vi "CLD 1 Elapsed Time Express Front Panel.vi"() -> ()   [LabVIEW 2009]
doc: "LabVIEW CLD-Übung 1"
panel:
  out "Fehler (Ausgang)":errorcluster
  in  "Fehler (Eingang)":errorcluster
  out "Verstrichene Zeit":string
  out "Zeit ist verstrichen":bool
  in  "Autom. zurücksetzen":bool
  in  "Zurücksetzen-Schaltfläche":bool
  in  "VI anhalten":bool
  in  "Zielzeit (s)":dbl
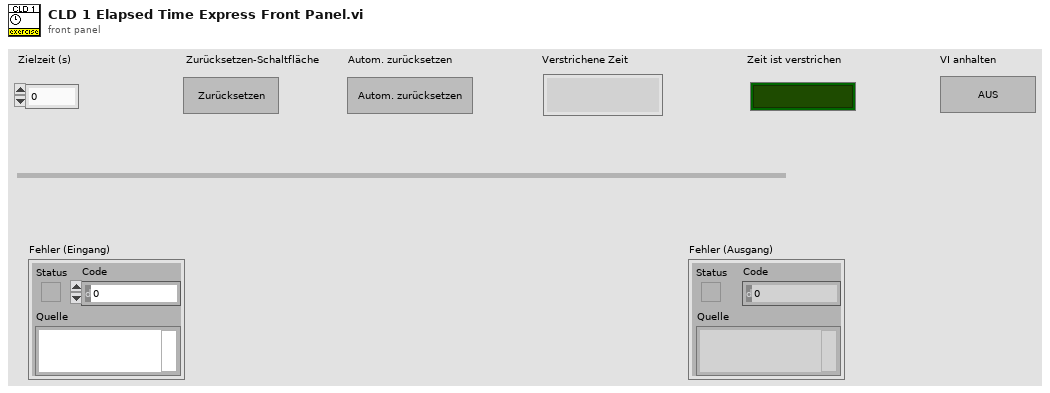
[diagram p1: front panel]
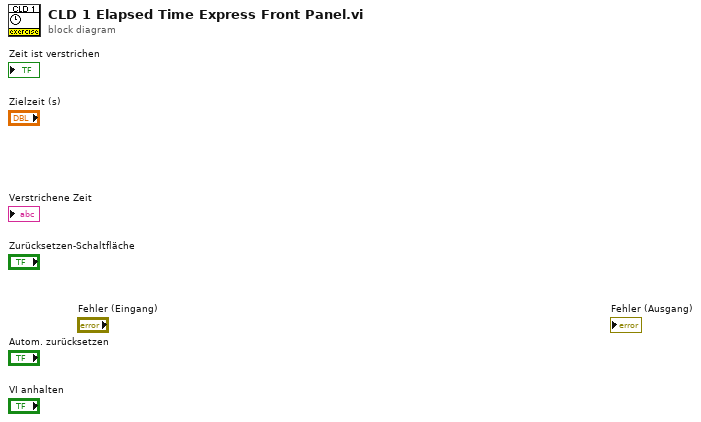
[diagram p0: block diagram]
diagram:
